vi "AT901 Transformation.vi"() -> ()   [LabVIEW 2017]
uses:
  AT901 API/Structures/Struct CallTrafo.ctl
  AT901 API/TypeDefinitions/ES_MeasMode.ctl
  AT901 API/Structures/Struct TransformationPoint.ctl
panel:
  out "CallTrafo":T1
  in  "CallTransformation":bool
  in  "Add Actual Point":bool
  out "Actual Point":dbl[](array[numeric])
  in  "Measure Actual Point":bool
  in  "stop":bool
  in  "Add Nominal Point":bool
  out "Actual Points (Measured)":dbl[][](array[numeric])
  out "Nominal Points":dbl[][](array[numeric])
  out "error out":errorcluster
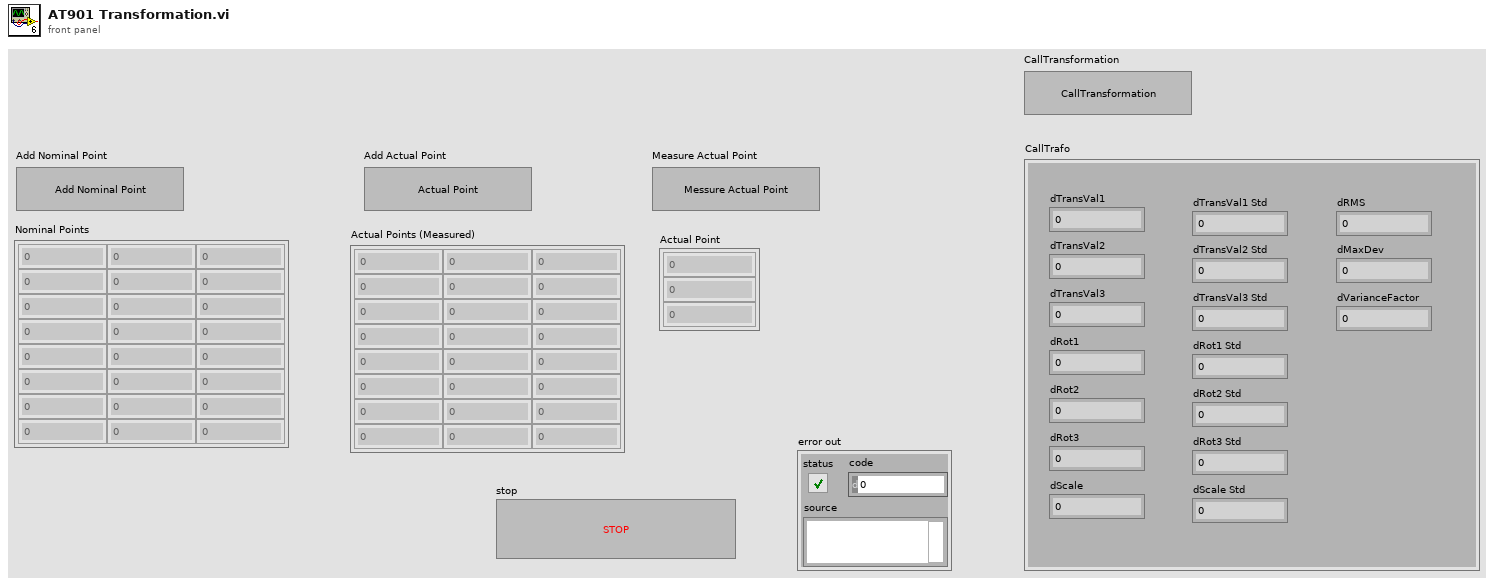
[diagram p1: front panel]
types:
  T1 = typedef "Struct CallTrafo.ctl" = cluster{"dTransVal1":dbl, "dTransVal2":dbl, "dTransVal3":dbl, "dRot1":dbl, "dRot2":dbl, "dRot3":dbl, "dScale":dbl, "dTransVal1 Std":dbl, "dTransVal2 Std":dbl, "dTransVal3 Std":dbl, "dRot1 Std":dbl, "dRot2 Std":dbl, "dRot3 Std":dbl, "dScale Std":dbl, "dRMS":dbl, "dMaxDev":dbl, "dVarianceFactor":dbl}
  T2 = typedef "ES_MeasMode.ctl" = enum32{"ES_MM_Stationary", "ES_MM_ContinuousTime", "ES_MM_ContinuousDistance", "ES_MM_Grid", "ES_MM_SphrereCenter", "ES_MM_CircleCenter", "ES_MM_6DStationary", "ES_MM_6DContinuousTime", "ES_MM_6DContinuousDistance", "ES_MM_6DGrid", "ES_MM_6DSphrereCenter", "ES_MM6DCircleCenter"}
  T3 = typedef "Struct TransformationPoint.ctl" = cluster{"dVal1":dbl, "dVal2":dbl, "dVal3":dbl, "dStd1":dbl, "dStd2":dbl, "dStd3":dbl, "dCovar12":dbl, "dCovar13":dbl, "dCovar23":dbl}
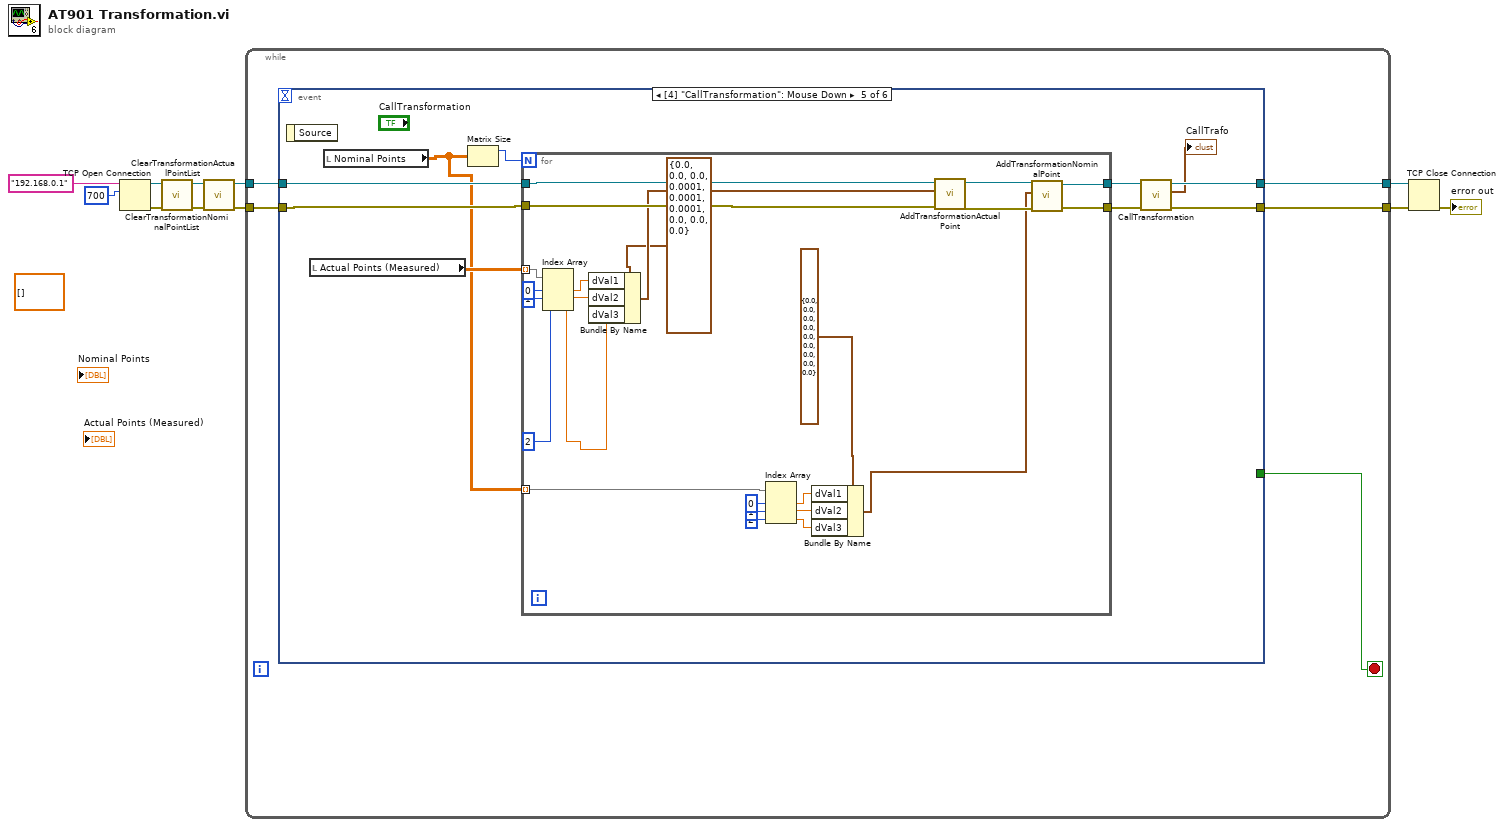
[diagram p0: block diagram]
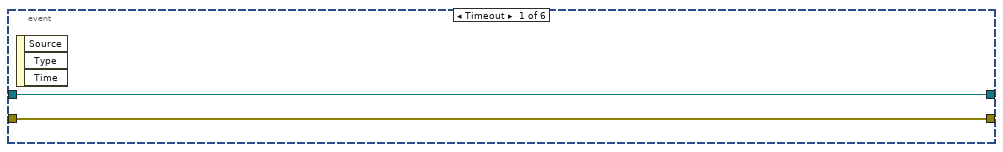
[diagram p2: hidden frame]
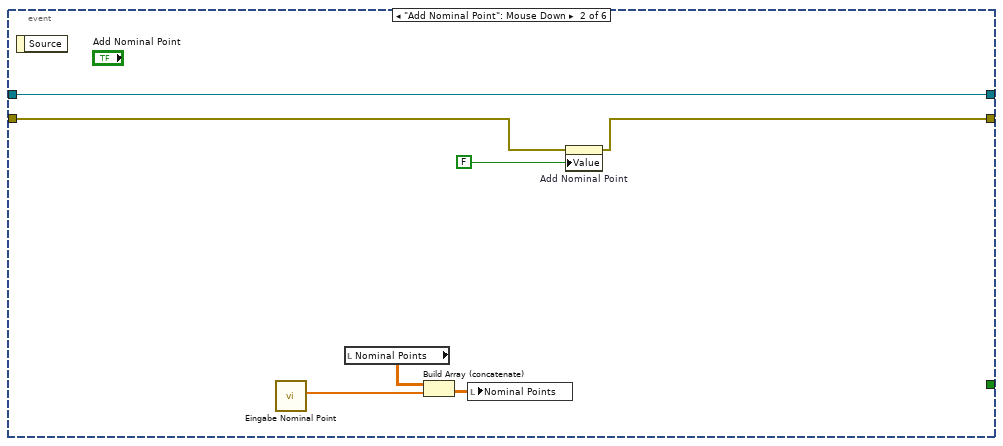
[diagram p3: hidden frame]
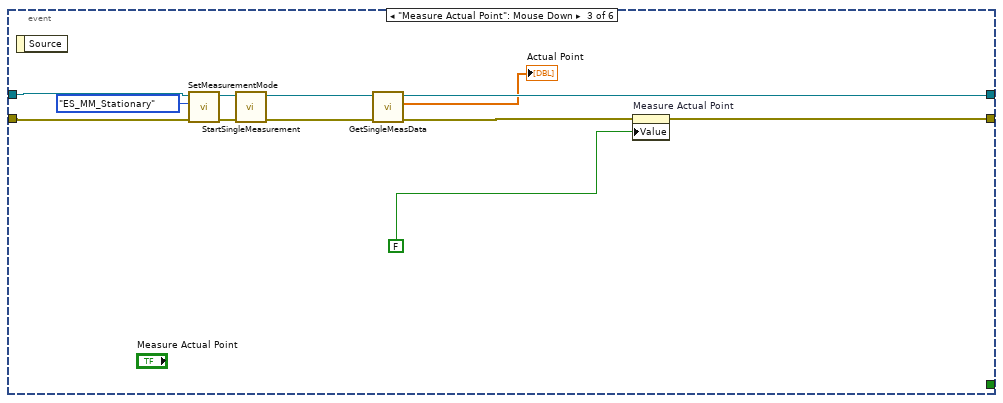
[diagram p4: hidden frame]
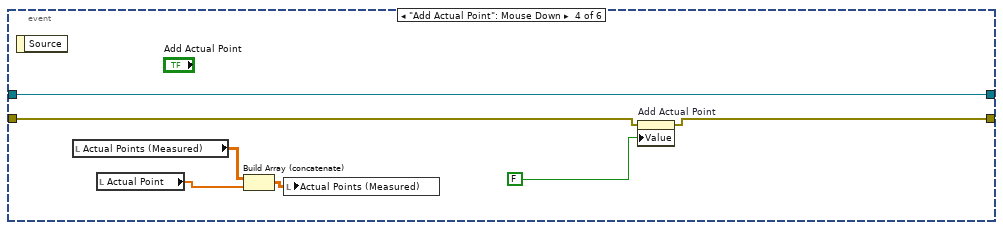
[diagram p5: hidden frame]
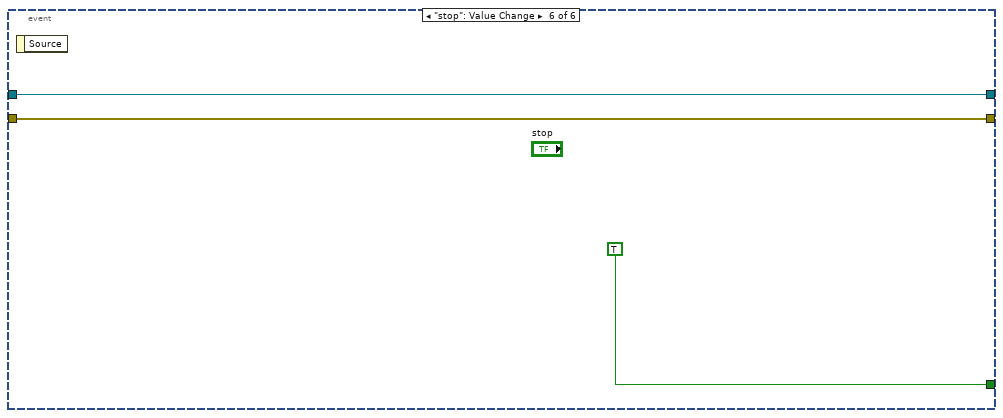
[diagram p6: hidden frame]
diagram:
  (unwired) dbl[][] [] ("Nominal Points")
  n1 = TCP Open Connection(address="192.168.0.1", remote port or service name=u16 700) -> (connection ID=w9:refnum<k5>, error out=w8:errorcluster)  [unwired: 3 in]
  n2 = call "ClearTransformationNominalPointList.vi"("error in (no error)"=w8, "TCP Network Connection in"=w9) -> ("error out"=w6:errorcluster, "TCP Network Connection out"=w7:refnum<k5>)  [unwired: 6 in, 2 out]
  n3 = call "ClearTransformationActualPointList.vi"("error in (no error)"=w6, "TCP Network Connection in"=w7) -> ("error out"=w2:errorcluster, "TCP Network Connection out"=w3:refnum<k5>)  [unwired: 6 in, 2 out]
  n4 = while {
    tunnel: [w16] -> w4
    tunnel: w3 -> [w15]
    tunnel: w2 -> [w14]
    tunnel: [w13] -> w1
    stop <- w12 stop-if-true
    n5 = event shown="[4] \"CallTransformation\": Mouse Down" {
      selector: _ -> [_ _ _ _ _ _]
      dyn-events: _ -> [_ _ _ _ _ _]
      timeout: _ -> [_ _ _ _ _ _]
      tunnel: [w18 w25 w30 w44 w47 w79] -> w16
      tunnel: w15 -> [w18 w25 w32 w44 w53 w79]
      tunnel: w14 -> [w17 w21 w31 w41 w52 w80]
      tunnel: [w17 w20 w26 w42 w46 w80] -> w13
      tunnel: [_ _ _ _ _ TRUE] -> w12
      event Timeout {
        n6 = event-data() -> ()  [unwired: 1 in, 3 out]
      }
      event "Add Nominal Point": Mouse Down {
        n7 = event-data() -> ()  [unwired: 1 in, 1 out]
        n8 = call "Eingabe Nominal Point.vi"() -> ("Array"=w23:dbl[])  [unwired: 11 in]
        n9 = local read "Nominal Points"() -> (w24:dbl[][])
        n10 = Build Array (concatenate)(w24, w23) -> (w19:dbl[][])
        n11 = local write "Nominal Points"(w19) -> ()
        n12 = property on="Add Nominal Point" class="Bool (strict)"(error in=w21, "Value"=FALSE ("Add Nominal Point")) -> (error out=w20:errorcluster)  [unwired: 1 in, 1 out]
      }
      event "Measure Actual Point": Mouse Down {
        n13 = event-data() -> ()  [unwired: 1 in, 1 out]
        n14 = call "SetMeasurementMode.vi"("error in (no error)"=w31, "ES_MeasMode"=ES_MeasMode."ES_MM_Stationary", "TCP Network Connection in"=w32) -> ("error out"=w36:errorcluster, "TCP Network Connection out"=w35:refnum<k5>)  [unwired: 5 in, 2 out]
        n15 = call "StartSingleMeasurement.vi"("error in (no error)"=w36, "TCP Network Connection in"=w35) -> ("error out"=w37:errorcluster, "TCP Network Connection out"=w34:refnum<k5>)  [unwired: 7 in, 1 out]
        n16 = call "GetSingleMeasData.vi"("error in (no error)"=w37, "TCP Network Connection in"=w34) -> ("error out"=w27:errorcluster, "Meas Result"=→"Actual Point":dbl[], "TCP Network Connection out"=w30:refnum<k5>)  [unwired: 6 in, 1 out]
        n17 = property on="Measure Actual Point" class="Bool (strict)"(error in=w27, "Value"=FALSE ("Messe Einzelpunkt")) -> (error out=w26:errorcluster)  [unwired: 1 in, 1 out]
      }
      event "Add Actual Point": Mouse Down {
        n18 = event-data() -> ()  [unwired: 1 in, 1 out]
        n19 = local read "Actual Points (Measured)"() -> (w39:dbl[][])
        n20 = local read "Actual Point"() -> (w40:dbl[])
        n21 = Build Array (concatenate)(w39, w40) -> (w38:dbl[][])
        n22 = local write "Actual Points (Measured)"(w38) -> ()
        n23 = property on="Add Actual Point" class="Bool (strict)"(error in=w41, "Value"=FALSE ("Add Actual Point")) -> (error out=w42:errorcluster)  [unwired: 1 in, 1 out]
      }
      event "CallTransformation": Mouse Down {
        n24 = event-data() -> ()  [unwired: 1 in, 1 out]
        n25 = local read "Actual Points (Measured)"() -> (w51:dbl[][])
        n26 = local read "Nominal Points"() -> (w50:dbl[][])
        n27 = Matrix Size(0:w50) -> (1:w54:i32)  [unwired: 1 out]
        n28 = for {
          N: w54 -> [_]
          tunnel: w53 -> [w78]
          tunnel: w52 -> [w77]
          tunnel: [w74] -> w49
          tunnel: [w73] -> w48
          tunnel: w51 -> [w72] mode=indexing
          tunnel: w50 -> [w58] mode=indexing
          n29 = Index Array(array=w72, index #1=0 ("index"), index #2=1 ("index"), index #3=2 ("index")) -> (element #1=w68:dbl, element #2=w67:dbl, element #3=w66:dbl)
          n30 = Bundle By Name(cluster=T3 {"dVal1"=0.0, "dVal2"=0.0, "dVal3"=0.0, "dStd1"=0.0001, "dStd2"=0.0001, "dStd3"=0.0001, "dCovar12"=0.0, "dCovar13"=0.0, "dCovar23"=0.0} ("Transformation Point"), "dVal1"=w68, "dVal2"=w67, "dVal3"=w66) -> (w65:T3)
          n31 = Index Array(array=w58, index #1=0 ("index"), index #2=1 ("index"), index #3=2 ("index")) -> (element #1=w61:dbl, element #2=w60:dbl, element #3=w59:dbl)
          n32 = Bundle By Name(cluster=T3 {"dVal1"=0.0, "dVal2"=0.0, "dVal3"=0.0, "dStd1"=0.0, "dStd2"=0.0, "dStd3"=0.0, "dCovar12"=0.0, "dCovar13"=0.0, "dCovar23"=0.0} ("Transformation Point"), "dVal1"=w61, "dVal2"=w60, "dVal3"=w59) -> (w57:T3)
          n33 = call "AddTransformationActualPoint.vi"("error in (no error)"=w77, "Transformation Point"=w65, "TCP Network Connection in"=w78) -> ("error out"=w75:errorcluster, "TCP Network Connection out"=w76:refnum<k5>)  [unwired: 5 in, 2 out]
          n34 = call "AddTransformationNominalPoint.vi"("error in (no error)"=w75, "Transformation Point"=w57, "TCP Network Connection in"=w76) -> ("error out"=w73:errorcluster, "TCP Network Connection out"=w74:refnum<k5>)  [unwired: 5 in, 2 out]
        }
        n35 = call "CallTransformation.vi"("error in (no error)"=w48, "TCP Network Connection in"=w49) -> ("error out"=w46:errorcluster, "CallTrafoCluster"=→"CallTrafo":T1, "TCP Network Connection out"=w47:refnum<k5>)  [unwired: 5 in, 2 out]
      }
      event "stop": Value Change {
        n36 = event-data() -> ()  [unwired: 1 in, 1 out]
      }
    }
  }
  n37 = TCP Close Connection(connection ID=w4, error in (no error)=w1) -> (error out=→"error out":errorcluster)  [unwired: 1 in, 1 out]
